vi "Add Row.vi"(6 "color":u32(colorbox)=16777215, 8 "error in":errorcluster, 9 "text":string, 10 "length":i32, 11 "XLS in":refnum<class "XLS.lvclass">=refnum) -> (0 "error out":errorcluster, 3 "XLS out":refnum<class "XLS.lvclass">)   [LabVIEW 2017, in "Report_lib.lvlib" / "XLS.lvclass"]
doc: "This method add colored row with some text\nin previously defined coordinates"
uses:
  XLS.lvclass
  <vilib>/Utility/NIReport.llb/Excel/NI_Excel.lvclass
  <vilib>/Utility/NIReport.llb/NI_report.lvclass
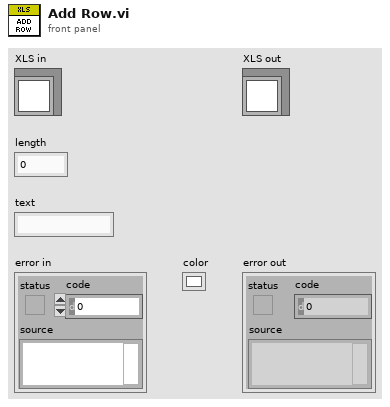
[diagram p1: front panel]
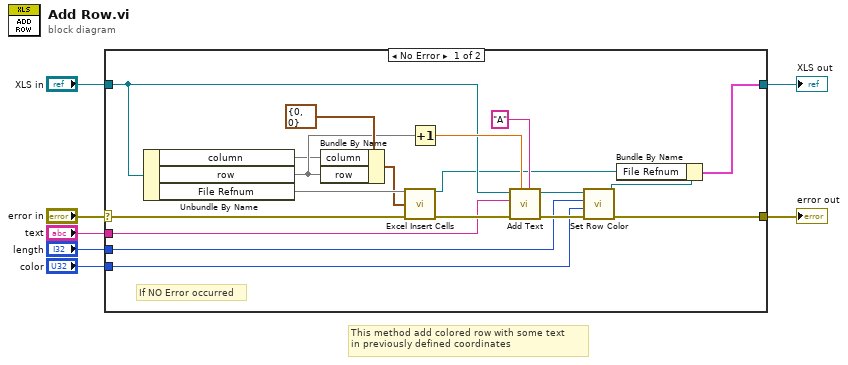
[diagram p0: block diagram]
diagram:
  # "This method add colored row with some text\nin previously defined coordinates"
  n1 = case shown="No Error" "error in" {
    selector: "error in" -> [w23 w28]
    tunnel: [w13 w28] -> w6
    tunnel: [w12 w27] -> w4
    tunnel: "XLS in" -> [w18 w27]
    tunnel: "text" -> [w11 _]
    tunnel: "length" -> [w10 _]
    tunnel: "color" -> [w9 _]
    frame No Error {
      # "If NO Error occurred"
      n2 = Unbundle By Name(w18) -> ("column"=w8, "row"=w21, "File Refnum"=w26)
      n3 = Bundle By Name(cluster=cluster{"row":i32, "column":i32} {"row"=0, "column"=0} ("start (0, 0)"), "column"=w8, "row"=w21) -> (w24:cluster{"row":i32, "column":i32})
      n4 = call <vilib>:"Excel Insert Cells.vi"("report in"=w26, "start (0, 0)"=w24, "error in (no error)"=w23) -> ("report out"=w14:refnum<class "NI_report.lvclass">, "error out"=w22:errorcluster)  [unwired: 11 in]
      n5 = Increment(x=w21) -> (x+1=w20:dbl)
      n6 = call "Add Text.vi"("Adr"="A", "Index"=w20, "error in"=w22, "text"=w11, "XLS in"=w18) -> ("error out"=w17:errorcluster, "XLS out"=w16:refnum<class "XLS.lvclass">)  [unwired: 5 in]
      n7 = call "Set Row Color.vi"("error in"=w17, "color"=w9, "length"=w10, "XLS in"=w16) -> ("error out"=w13:errorcluster, "XLS out"=w15:refnum<class "XLS.lvclass">)  [unwired: 6 in]
      n8 = Bundle By Name(cluster=w15, "File Refnum"=w14) -> (w12:cluster{})
    }
    frame Error {
    }
  }
  "error out" <- w6
  "XLS out" <- w4
